vi "IDN.vi"(8 "error in (no error)":errorcluster, 11 "VISA resource name":refnum<visa-resource-name>) -> (0 "error out":errorcluster, 2 "*IDN?":string, 3 "VISA Refnum out":refnum<visa-resource-name>)   [LabVIEW 2016, in "RP100.lvclass"]
uses:
  RP100.lvclass
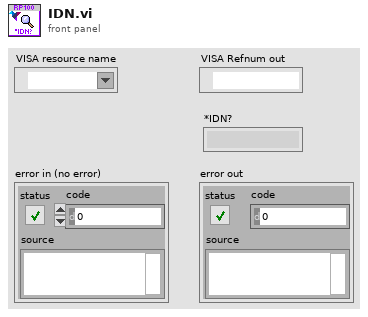
[diagram p1: front panel]
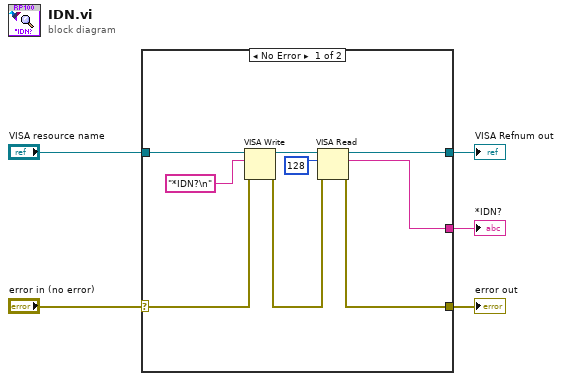
[diagram p0: block diagram]
diagram:
  n1 = case shown="No Error" "error in (no error)" {
    selector: "error in (no error)" -> [w7 w16]
    tunnel: [w14 w15] -> w5
    tunnel: "VISA resource name" -> [w13 w15]
    tunnel: [w9 w16] -> w3
    tunnel: [w8 _] -> w2
    frame No Error {
      n2 = VISA Write(VISA resource name=w13, write buffer="*IDN?\n" ("format string"), error in (no error)=w7) -> (VISA resource name out=w10:refnum<visa-resource-name>, error out=w12:errorcluster)  [unwired: 1 out]
      n3 = VISA Read(VISA resource name=w10, byte count=u32 128, error in (no error)=w12) -> (VISA resource name out=w14:refnum<visa-resource-name>, read buffer=w8:string, error out=w9:errorcluster)  [unwired: 1 out]
    }
    frame Error {
    }
  }
  "*IDN?" <- w2
  "VISA Refnum out" <- w5
  "error out" <- w3
